vi "Analog Continous Output.vi"() -> ()   [LabVIEW 2009, in "MicroDAQ.lvlib"]
doc: "This example demonstrates how to continuously re-generate analog output data from a buffer in your computer's memory.\n\nRefer to your device documentation for pinouts and hardware capabilities."
uses:
  <instrlib>/MicroDAQ/MicroDAQ.lvlib
  <instrlib>/MicroDAQ/Tools/Analog Channel Enum.ctl
  <instrlib>/MicroDAQ/Tools/Analo Range Enum.ctl
  <instrlib>/MicroDAQ/Tools/Encoder type.ctl
  <instrlib>/MicroDAQ/Tools/Trigger Encoder condition enum.ctl
  <instrlib>/MicroDAQ/Tools/Trigger DIO ring.ctl
  <instrlib>/MicroDAQ/Tools/Analog mode.ctl
  <instrlib>/MicroDAQ/Channel/Analog Output/Write NChan NSamp 1D Waveform.vi
  <instrlib>/MicroDAQ/Channel/Analog Output/AO Configure Channel.vi
  <instrlib>/MicroDAQ/Channel/Analog Output/Triggering DIO state.vi
  <instrlib>/MicroDAQ/Channel/Analog Output/Triggering DIO Pattern.vi
  <instrlib>/MicroDAQ/Channel/Analog Output/Triggering Encoder.vi
  <instrlib>/MicroDAQ/Channel/Analog Output/Analog output.lvclass
  <vilib>/measure/NI_MABase.lvlib
panel:
  in  "Triggering":T1(tab)
  in  "Level":bool=TRUE
  in  "Pin":T2 items=["DIO1"=1, "DIO2"=2, "DIO3"=3, "DIO4"=4, "DIO5"=5, "DIO6"=6, "DIO7"=7, "DIO8"=8]
  in  "Pattern":string
  in  "Channel":T3 items=["ENC1"=1, "ENC2"=2]
  in  "Condition":T4
  in  "Position":i32
  in  "Waveforms":T5(array[cluster])=[{"Waveform Type"=enum."Sine Wave", "Amplitude"=1.0, "Frequency"=10.0}] {"Frequency" format="%0.2p"; "Amplitude" format="%0.2p"}
  in  "Stop":bool
  out "Waveform Graph":waveform(dbl)[](graph)=[{"t0"=timestamp(0 s since 1904-01-01), "dt"=0.001, "Y"=[]}]
  in  "Sample Rate":dbl=1000.0 format="%#_13g"
  in  "Ranges":T6[](array[typedef])=[enum."±10V"]
  in  "Physical channels":T7[](array[typedef])=[enum."AO1"]
  in  "IP address":string="10.10.1.1"
  # "Device settings"
  # "Signal Settings"
  # "Output"
  # "Channel Settings"
  # "The number of elements in the waveform array must equal the number of channels and Ranges."
  # "Mode and Timing Settings"
  # "Tip: x->ignored, 1->HI, 0->LOW\nexampe: 11xxxxxx\nmore info in Triggering VI help"
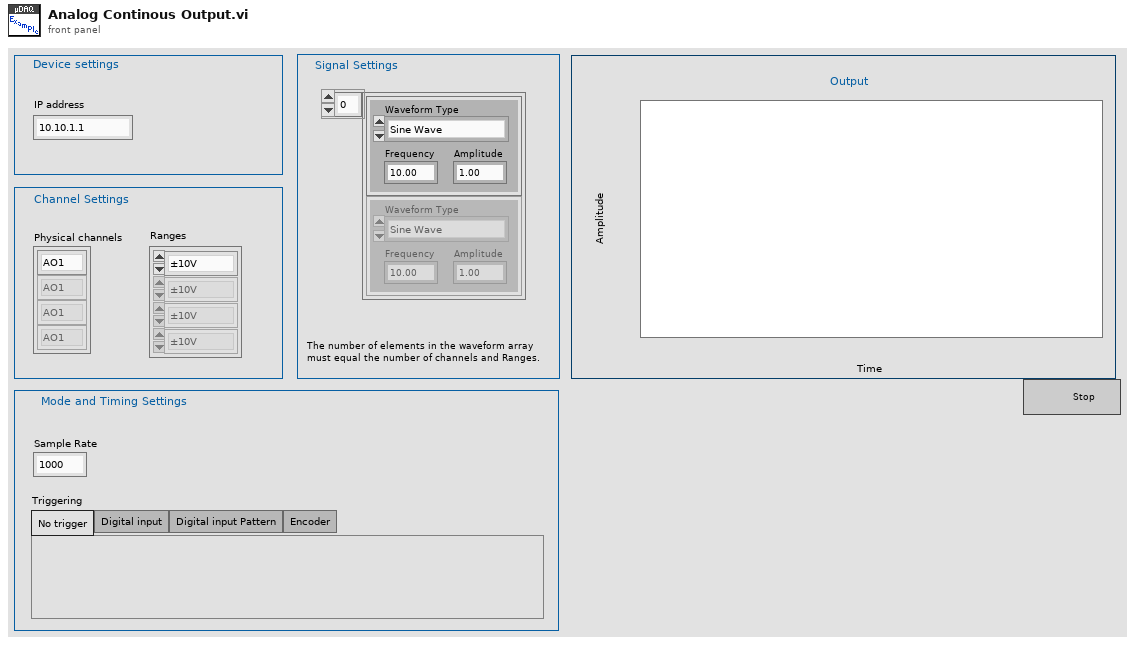
[diagram p1: front panel]
types:
  T1 = enum32{"No trigger", "Digital input", "Digital input Pattern", "Encoder"}
  T2 = typedef "MicroDAQ.lvlib/Trigger DIO ring.ctl" = u16
  T3 = typedef "MicroDAQ.lvlib/Encoder type.ctl" = u8
  T4 = typedef "MicroDAQ.lvlib/Trigger Encoder condition enum.ctl" = enum16{"Lower then", "Greater then"}
  T5 = cluster{"Waveform Type":enum16{"Sine Wave", "Triangle Wave", "Square Wave", "Sawtooth Wave"}, "Amplitude":dbl, "Frequency":dbl}[]
  T6 = typedef "MicroDAQ.lvlib/Analo Range Enum.ctl" = enum16{"±10V", "0-10V", "±5V", "0-5V", "±5.12V", "±2.56V", "±2.5V", "±2V", "±1.24V", "±0.64V"}
  T7 = typedef "MicroDAQ.lvlib/Analog Channel Enum.ctl" = enum16{"None", "AO1", "AO2", "AO3", "AO4", "AO5", "AO6", "AO7", "AO8", "AO9", "AO10", "AO11", "AO12", "AO13", "AO14", "AO15", "AO16"}
  T8 = typedef "MicroDAQ.lvlib/Analog mode.ctl" = enum16{"Periodic", "Stream"}
  T9 = enum16{"Sine Wave", "Triangle Wave", "Square Wave", "Sawtooth Wave"}
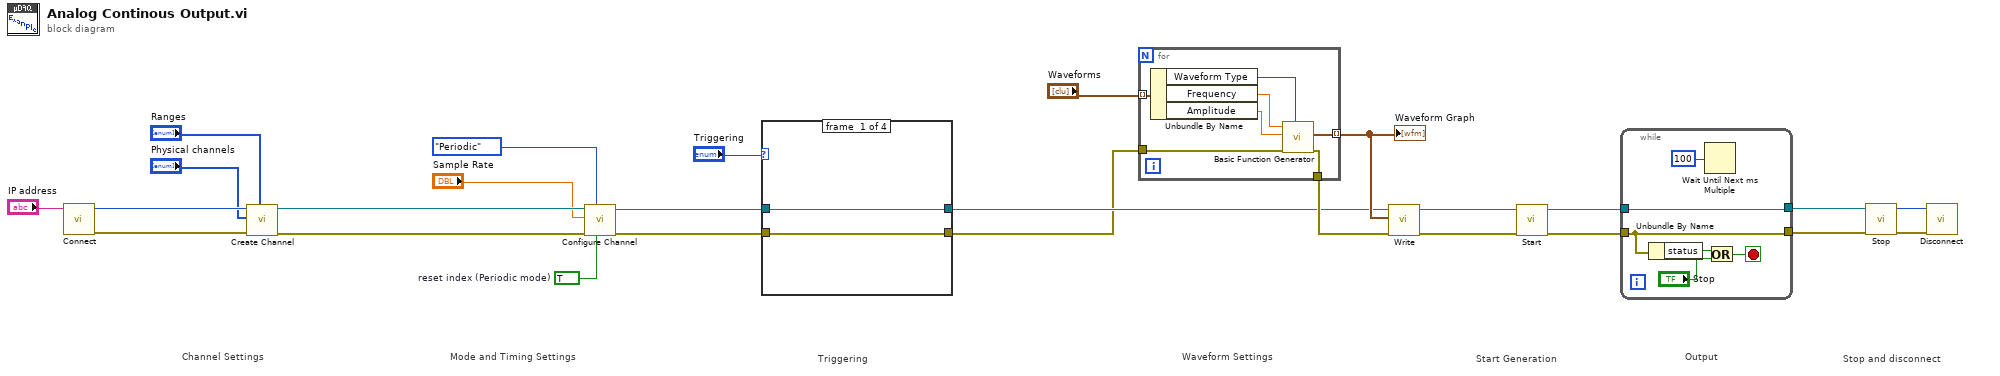
[diagram p0: block diagram]
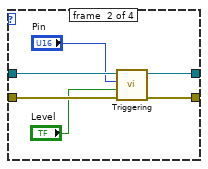
[diagram p2: hidden frame]
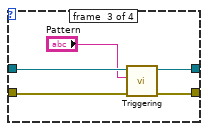
[diagram p3: hidden frame]
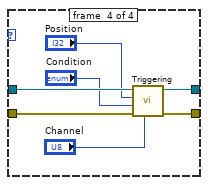
[diagram p4: hidden frame]
diagram:
  w11 = TRUE  # reset index (Periodic mode)
  # "Triggering"
  # "Start Generation"
  # "Stop and disconnect"
  # "Output"
  # "Waveform Settings"
  # "Mode and Timing Settings"
  # "Channel Settings"
  n1 = call <instrlib>:"Connect.vi"("IP address"="IP address") -> ("error out"=w25:errorcluster, "connection ID"=w26:i32)  [unwired: 9 in]
  n2 = call-poly <instrlib>:"Create Channel.vi"("Ranges"="Ranges", "error in (no error)"=w25, "Phisical channels"="Physical channels", "Connection ID"=w26) -> ("error out"=w20:errorcluster, "Task Out"=w21:refnum<class "Analog output.lvclass">)  [unwired: 6 in]
  n3 = call-poly <instrlib>:"Configure Channel.vi"("Reset index (Periodic mode)"=w11, "Mode"=Analog_mode."Periodic" ("mode"), "error in (no error)"=w20, "Sample rate"="Sample Rate", "Analog Output in"=w21) -> ("error out"=w3:errorcluster, "Analog Output out"=w4:refnum<class "Analog output.lvclass">)  [unwired: 5 in]
  n4 = case shown="\"Digital input\"" "Triggering" {
    tunnel: w4 -> [w28 w34 w37 w44]
    tunnel: [w28 w33 w39 w46] -> w2
    tunnel: w3 -> [w27 w32 w36 w43]
    tunnel: [w27 w31 w38 w45] -> w1
    frame #0 {
    }
    frame #1 {
      n5 = call-poly <instrlib>:"Triggering.vi"("error in (no error)"=w32, "level"="Level", "pin"="Pin", "MicroDAQ.lvlib:Analog output.lvclass"=w34) -> ("error out"=w31:errorcluster, "MicroDAQ.lvlib:Analog output.lvclass out"=w33:refnum<class "Analog output.lvclass">)  [unwired: 6 in]
    }
    frame #2 {
      n6 = call-poly <instrlib>:"Triggering.vi"("error in (no error)"=w36, "pattern"="Pattern", "MicroDAQ.lvlib:Analog output.lvclass"=w37) -> ("error out"=w38:errorcluster, "MicroDAQ.lvlib:Analog output.lvclass out"=w39:refnum<class "Analog output.lvclass">)  [unwired: 7 in]
    }
    frame #3 {
      n7 = call-poly <instrlib>:"Triggering.vi"("Channel (1|2)"="Channel", "error in (no error)"=w43, "condition"="Condition", "position"="Position", "MicroDAQ.lvlib:Analog output.lvclass"=w44) -> ("error out"=w45:errorcluster, "MicroDAQ.lvlib:Analog output.lvclass out"=w46:refnum<class "Analog output.lvclass">)  [unwired: 5 in]
    }
  }
  n8 = for {
    tunnel: [w53] -> w8
    tunnel: "Waveforms" -> [w52] mode=indexing
    tunnel: [w48] -> w9 mode=indexing
    tunnel: w1 -> [w47]
    n9 = Unbundle By Name(w52) -> ("Waveform Type"=w51:T9, "Frequency"=w50:dbl, "Amplitude"=w49:dbl)
    n10 = call <vilib>:"Basic Function Generator.vi"("signal type"=w51, "error in (no error)"=w47, "amplitude"=w49, "frequency"=w50) -> ("error out"=w53:errorcluster, "signal out"=w48:waveform(dbl))  [unwired: 5 in, 1 out]
  }
  "Waveform Graph" <- w9
  n11 = call-poly <instrlib>:"Write.vi"("error in (no error)"=w8, "data"=w9, "Analog Output in"=w2) -> ("error out"=w6:errorcluster, "Analog Output out"=w7:refnum<class "Analog output.lvclass">)  [unwired: 7 in]
  n12 = call-dynamic "Start.vi"("error in (no error)"=w6, "Analog Output in"=w7) -> ("error out"=w17:errorcluster, "Analog Output out"=w18:refnum<class "Analog output.lvclass">)  [unwired: 8 in]
  n13 = while {
    tunnel: w18 -> [w57]
    tunnel: w17 -> [w59]
    tunnel: [w59] -> w15
    tunnel: [w57] -> w16
    stop <- w55 stop-if-true
    n14 = Unbundle By Name(w59) -> ("status"=w54:bool)
    n15 = Wait Until Next ms Multiple(millisecond multiple=u32 100) -> ()  [unwired: 1 out]
    n16 = Or(x=w54, y="Stop") -> (x .or. y?=w55:bool)
  }
  n17 = call-dynamic "Stop.vi"("error in (no error)"=w15, "Analog Output in"=w16) -> ("error out"=w13:errorcluster, "connection ID"=w14:i32)  [unwired: 8 in]
  n18 = call <instrlib>:"Disconnect.vi"("error in (no error)"=w13, "connection ID"=w14) -> ()  [unwired: 9 in, 1 out]
